vi "__FilterSet_ParamChange.vi"(0 "Param in":cluster{"mode":u8, "AccCode":u32, "AccMask":u32}, 5 "CtrlRef":T1, 7 "IDRef":refnum<vi>[](array[refnum]), 9 "EIDRef":refnum<vi>[](array[refnum]), 11 "error in (no error)":errorcluster, 12 "IDRef 2":refnum<vi>[](array[refnum]), 13 "EIDRef 2":refnum<vi>[](array[refnum])) -> (4 "Param out":cluster{"mode":u8, "AccCode":u32, "AccMask":u32}, 15 "error out":errorcluster)   [LabVIEW 2011]
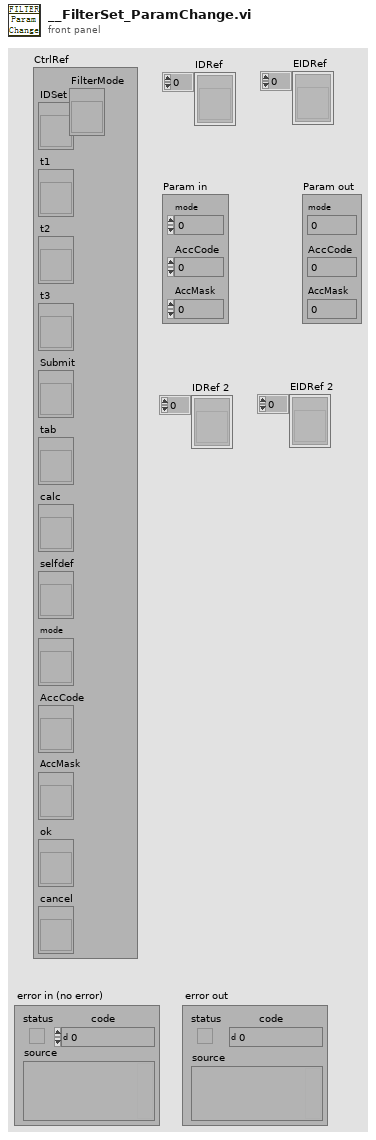
[diagram p1: front panel]
types:
  T1 = cluster{"FilterMode":refnum<vi>, "IDSet":refnum<vi>, "t1":refnum<vi>, "t2":refnum<vi>, "t3":refnum<vi>, "Submit":refnum<vi>, "tab":refnum<vi>, "calc":refnum<vi>, "selfdef":refnum<vi>, "mode":refnum<vi>, "AccCode":refnum<vi>, "AccMask":refnum<vi>, "ok":refnum<vi>, "cancel":refnum<vi>}
  T2 = enum16{"接收所有数据", "标准帧滤波（设定接收单个ID）", "扩展帧滤波（设定接收单个ID）", "标准帧滤波（仅ID，自由设定）", "扩展帧滤波（仅ID，自由设定）"}
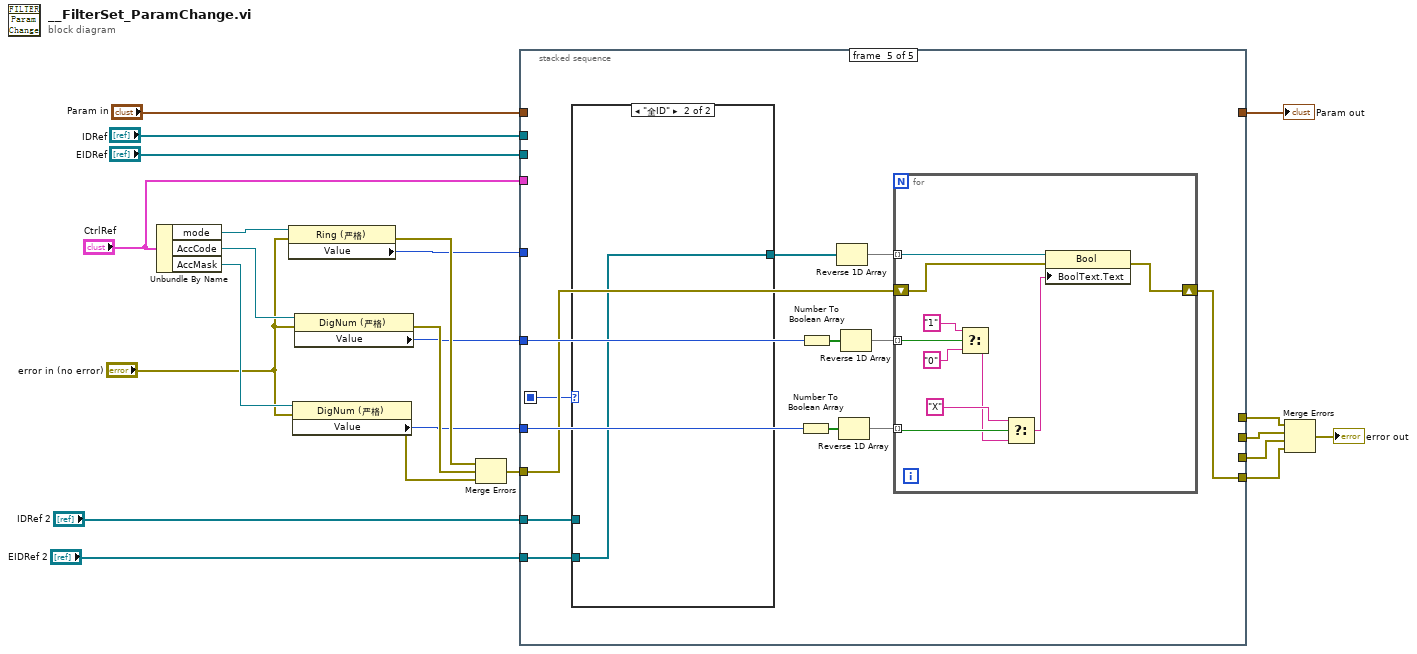
[diagram p0: block diagram]
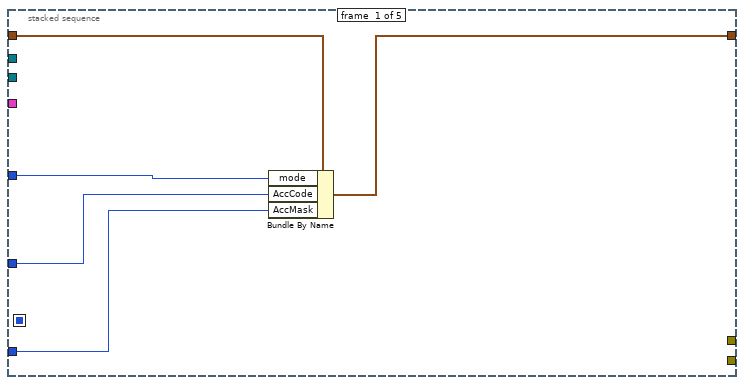
[diagram p2: hidden frame]
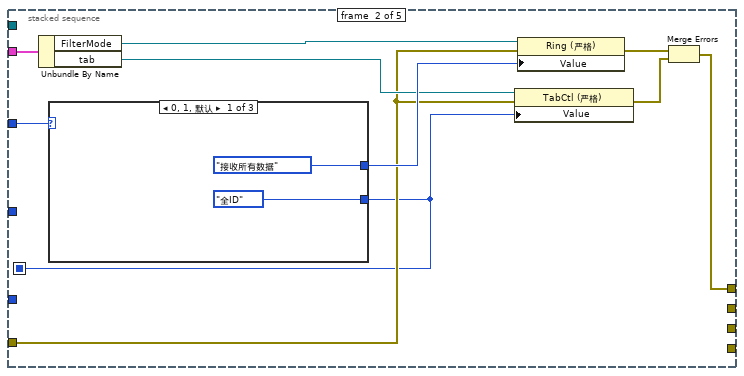
[diagram p3: hidden frame]
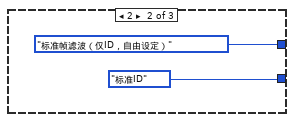
[diagram p4: hidden frame]
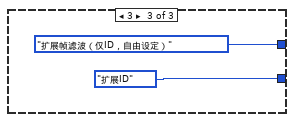
[diagram p5: hidden frame]
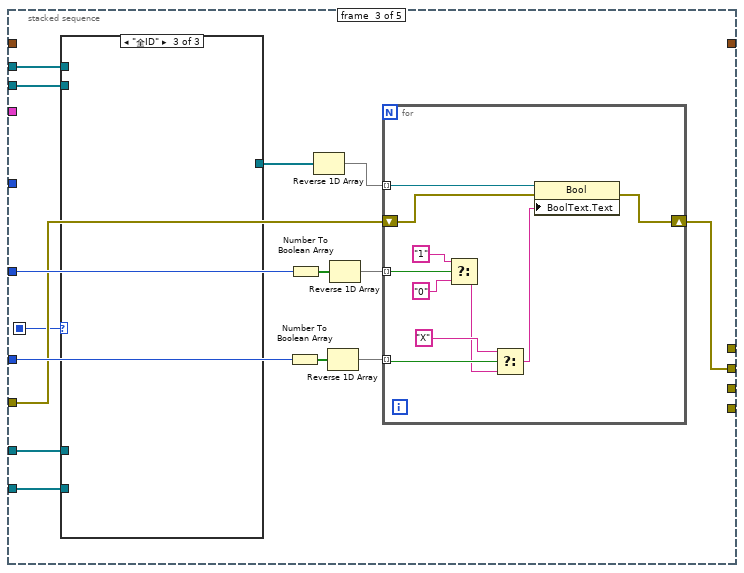
[diagram p6: hidden frame]
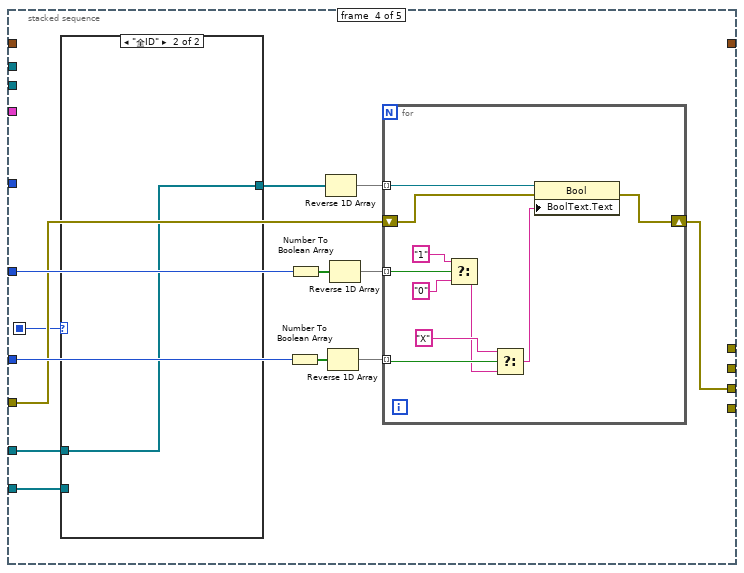
[diagram p9: hidden frame]
diagram:
  n1 = Unbundle By Name("CtrlRef") -> ("mode"=w23:refnum<vi>, "AccCode"=w22:refnum<vi>, "AccMask"=w21:refnum<vi>)
  n2 = property class="Ring (严格)"(reference=w23, error in="error in (no error)") -> (error out=w19:errorcluster, "Value"=w16:u8)  [unwired: 1 out]
  n3 = property class="DigNum (严格)"(reference=w21, error in="error in (no error)") -> (error out=w17:errorcluster, "Value"=w14:u32)  [unwired: 1 out]
  n4 = property class="DigNum (严格)"(reference=w22, error in="error in (no error)") -> (error out=w18:errorcluster, "Value"=w15:u32)  [unwired: 1 out]
  n5 = Merge Errors(w19, w18, w17) -> (w13:errorcluster)
  n6 = stacked-sequence {
    seq-local: [_ w29 _ _ _] -> [_ _ w50 w76 w100]
    tunnel: w16 -> [w27 w38 _ _ _]
    tunnel: w15 -> [w26 _ w58 w83 w107]
    tunnel: w14 -> [w25 _ w59 w84 w108]
    tunnel: w13 -> [_ w33 w57 w82 w106]
    tunnel: "Param in" -> [w28 _ _ _ _]
    tunnel: [w24 _ _ _ _] -> w11
    tunnel: "CtrlRef" -> [_ w37 _ _ _]
    tunnel: [_ w30 _ _ _] -> w8
    tunnel: "IDRef" -> [_ _ w47 _ _]
    tunnel: "EIDRef" -> [_ _ w45 _ _]
    tunnel: [_ _ w51 _ _] -> w7
    tunnel: "IDRef 2" -> [_ _ w49 w75 w99]
    tunnel: "EIDRef 2" -> [_ _ w48 w74 w98]
    tunnel: [_ _ _ w72 _] -> w2
    tunnel: [_ _ _ _ w96] -> w1
    frame #0 {
      n7 = Bundle By Name(cluster=w28, "mode"=w27, "AccCode"=w26, "AccMask"=w25) -> (w24:cluster{"mode":u8, "AccCode":u32, "AccMask":u32})
    }
    frame #1 {
      n8 = Unbundle By Name(w37) -> ("FilterMode"=w36:refnum<vi>, "tab"=w34:refnum<vi>)
      n9 = case shown="0, 1, 默认" w38 {
        tunnel: [T2."接收所有数据" ("值") T2."标准帧滤波（仅ID，自由设定）" ("值") T2."扩展帧滤波（仅ID，自由设定）" ("值")] -> w35
        tunnel: [enum32{"标准ID", "扩展ID", "全ID"}."全ID" ("tab") enum32{"标准ID", "扩展ID", "全ID"}."标准ID" ("tab") enum32{"标准ID", "扩展ID", "全ID"}."扩展ID" ("tab")] -> w29
        frame 0, 1, Default {
        }
        frame 2 {
        }
        frame 3 {
        }
      }
      n10 = property class="TabCtl (严格)"(reference=w34, error in=w33, "Value"=w29) -> (error out=w31:errorcluster)  [unwired: 1 out]
      n11 = property class="Ring (严格)"(reference=w36, error in=w33, "Value"=w35) -> (error out=w32:errorcluster)  [unwired: 1 out]
      n12 = Merge Errors(w32, w31) -> (w30:errorcluster)
    }
    frame #2 {
      n13 = case shown="\"全ID\"" w50 {
        tunnel: w49 -> [_ _ _]
        tunnel: w48 -> [_ _ _]
        tunnel: w47 -> [w60 _ _]
        tunnel: [w60 w61 _] -> w46
        tunnel: w45 -> [_ w61 _]
        frame "标准ID", Default {
        }
        frame "扩展ID" {
        }
        frame "全ID" {
        }
      }
      n14 = Number To Boolean Array(number=w59) -> (Boolean array=w54:bool[])
      n15 = Number To Boolean Array(number=w58) -> (Boolean array=w55:bool[])
      n16 = Reverse 1D Array(array=w46) -> (reversed array=w56:refnum<vi>[])
      n17 = Reverse 1D Array(array=w54) -> (reversed array=w53:bool[])
      n18 = Reverse 1D Array(array=w55) -> (reversed array=w52:bool[])
      n19 = for {
        tunnel: w56 -> [w70] mode=indexing
        tunnel: w53 -> [w71] mode=indexing
        tunnel: w52 -> [w66] mode=indexing
        shift-right: [w68] -> w51
        shift-left: w57 -> [w69]
        n20 = Select(t="1", s=w66, f="0") -> (s? t:f=w63:string)
        n21 = Select(t="X", s=w71, f=w63) -> (s? t:f=w62:string)
        n22 = property class="Bool"(reference=w70, error in=w69, "BoolText.Text"=w62) -> (error out=w68:errorcluster)  [unwired: 1 out]
      }
    }
    frame #3 {
      n23 = case shown="\"全ID\"" w76 {
        tunnel: w75 -> [_ w85]
        tunnel: w74 -> [_ _]
        tunnel: [_ w85] -> w73
        frame "标准ID", Default {
        }
        frame "全ID" {
        }
      }
      n24 = Number To Boolean Array(number=w84) -> (Boolean array=w79:bool[])
      n25 = Number To Boolean Array(number=w83) -> (Boolean array=w80:bool[])
      n26 = Reverse 1D Array(array=w73) -> (reversed array=w81:refnum<vi>[])
      n27 = Reverse 1D Array(array=w79) -> (reversed array=w78:bool[])
      n28 = Reverse 1D Array(array=w80) -> (reversed array=w77:bool[])
      n29 = for {
        tunnel: w81 -> [w94] mode=indexing
        tunnel: w78 -> [w95] mode=indexing
        tunnel: w77 -> [w90] mode=indexing
        shift-right: [w92] -> w72
        shift-left: w82 -> [w93]
        n30 = Select(t="1", s=w90, f="0") -> (s? t:f=w87:string)
        n31 = Select(t="X", s=w95, f=w87) -> (s? t:f=w86:string)
        n32 = property class="Bool"(reference=w94, error in=w93, "BoolText.Text"=w86) -> (error out=w92:errorcluster)  [unwired: 1 out]
      }
    }
    frame #4 {
      n33 = case shown="\"全ID\"" w100 {
        tunnel: w99 -> [_ _]
        tunnel: w98 -> [_ w109]
        tunnel: [_ w109] -> w97
        frame "标准ID", Default {
        }
        frame "全ID" {
        }
      }
      n34 = Number To Boolean Array(number=w108) -> (Boolean array=w103:bool[])
      n35 = Number To Boolean Array(number=w107) -> (Boolean array=w104:bool[])
      n36 = Reverse 1D Array(array=w97) -> (reversed array=w105:refnum<vi>[])
      n37 = Reverse 1D Array(array=w103) -> (reversed array=w102:bool[])
      n38 = Reverse 1D Array(array=w104) -> (reversed array=w101:bool[])
      n39 = for {
        tunnel: w105 -> [w118] mode=indexing
        tunnel: w102 -> [w119] mode=indexing
        tunnel: w101 -> [w114] mode=indexing
        shift-right: [w116] -> w96
        shift-left: w106 -> [w117]
        n40 = Select(t="1", s=w114, f="0") -> (s? t:f=w111:string)
        n41 = Select(t="X", s=w119, f=w111) -> (s? t:f=w110:string)
        n42 = property class="Bool"(reference=w118, error in=w117, "BoolText.Text"=w110) -> (error out=w116:errorcluster)  [unwired: 1 out]
      }
    }
  }
  "Param out" <- w11
  n43 = Merge Errors(w8, w7, w2, w1) -> (→"error out":errorcluster)
